vi "Get Magnet Field.vi"(4 "Axis":T1, 8 "error in (no error)":errorcluster, 11 "Instrument.Oxford1820 in":refnum<class "Instrument.Oxford1820.lvclass">) -> (0 "error out":errorcluster, 1 "Status":variant, 2 "B Field (T)":dbl, 3 "Instrument.Oxford1820 out":refnum<class "Instrument.Oxford1820.lvclass">)   [LabVIEW 2016, in "Instrument.Oxford1820.lvclass"]
uses:
  Instrument.Oxford1820.lvclass
  <userlib>/LevyLab/Levylab Instruments/Instrument Types/Cryostat/Typedefs/Magnet Axis--Enum.ctl
  <userlib>/LevyLab/Levylab Instruments/Instrument Types/Cryostat/Instrument.Cryostat.lvclass
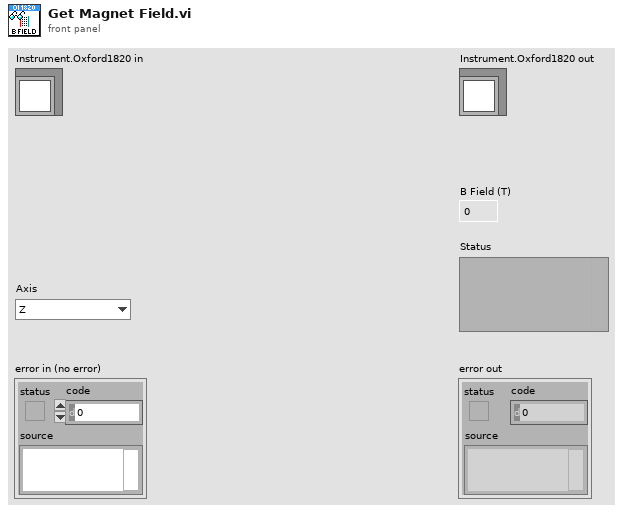
[diagram p1: front panel]
types:
  T1 = typedef "Instrument.Cryostat.lvclass/Magnet Axis--Enum.ctl" = enum16{"Z", "X", "Y"}
  T2 = typedef "Instrument.Oxford1820.lvclass/Status.ctl" = cluster{"Magnet Field":dbl, "PS Field":dbl, "Target Field":dbl, "Target Field Rate":dbl, "Voltage":dbl, "Current":dbl, "Switch":bool, "Mercury State":string}
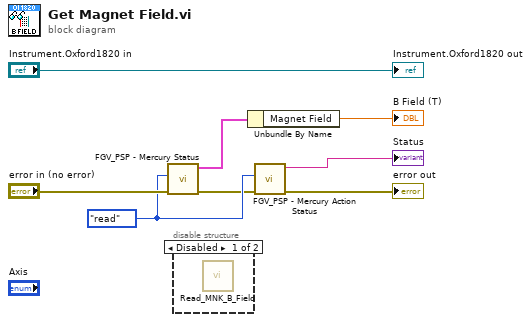
[diagram p0: block diagram]
diagram:
  w4 = enum16{"write", "read"}."read" ("Function")
  n1 = call "FGV_PSP - Mercury Status.vi"("error in"="error in (no error)", "Function"=w4) -> ("error out"=w3:errorcluster, "Status"=w6:T2)  [unwired: 4 in]
  n2 = disable-structure shown="Disabled" {
    frame Disabled {
      n3 = call "Read_MNK_B_Field.vi"() -> ()  [unwired: 9 in, 3 out]
    }
    frame Enabled {
    }
  }
  n4 = Unbundle By Name(w6) -> ("Magnet Field"=→"B Field (T)":dbl)
  n5 = call "FGV_PSP - Mercury Action Status.vi"("error in"=w3, "Function"=w4) -> ("error out"=→"error out":errorcluster, "Mercury Status 2"=→"Status":string)  [unwired: 4 in]
  "Instrument.Oxford1820 out" <- "Instrument.Oxford1820 in"
